vi "Corr Transducers To Meas Folder.vi"(8 "error in":errorcluster, 10 "measurement root path":path, 11 "transducers in":cluster{"channels":T1[], "last path":path} {"channels"."Phase index" min=1 step=1}) -> (0 "error out":errorcluster, 3 "transducers out":cluster{"channels":T1[], "last path":path} {"channels"."Phase index" min=1 step=1})   [LabVIEW 2013]
doc: "This VI will copy all transducer corrections to the measurement root path."
uses:
  Corr Tranducer Item.ctl
panel:
  # "ADC:"
  # "ADC:"
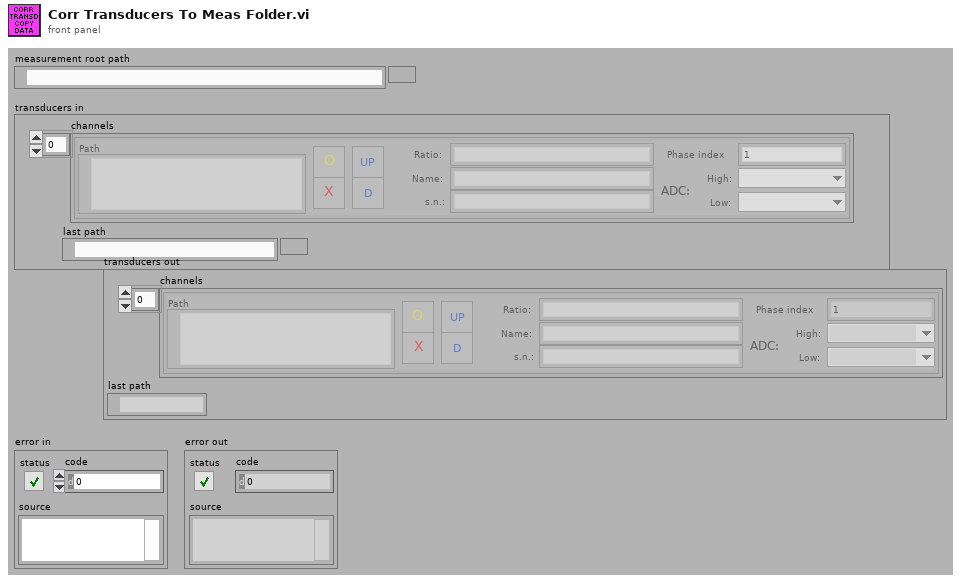
[diagram p1: front panel]
types:
  T1 = typedef "Corr Tranducer Item.ctl" = cluster{"Path":path, "Ratio:":string, "Name:":string, "btn rem":bool, "btn up":bool, "btn down":bool, "s.n.:":string, "btn open":bool, "ratio o/i":dbl, "chn hi":u16, "chn lo":u16, "Phase index":i32}
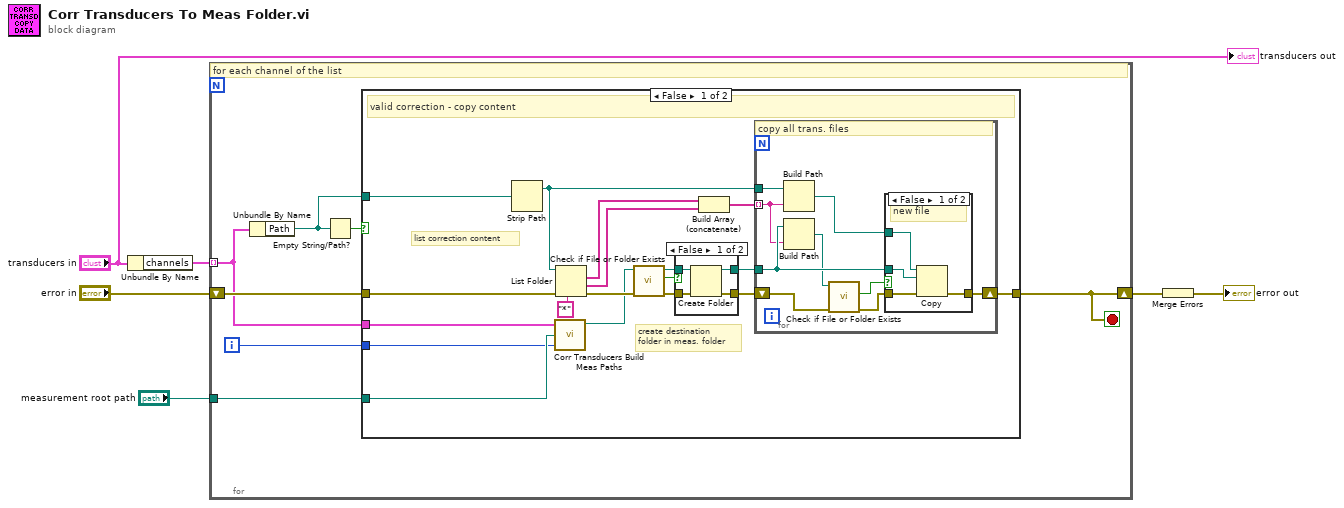
[diagram p0: block diagram]
diagram:
  n1 = Unbundle By Name("transducers in") -> ("channels"=w6:T1[])
  n2 = for {
    tunnel: w6 -> [w8] mode=indexing
    tunnel: "measurement root path" -> [w10]
    shift-right: [w9] -> w4
    shift-left: "error in" -> [w12]
    i -> [w7]
    stop <- w9 stop-if-true
    # "for each channel of the list"
    n3 = Unbundle By Name(w8) -> ("Path"=w11:path)
    n4 = Empty String/Path?(string/path=w11) -> (empty?=w13:bool)
    n5 = case shown="False" w13 {
      tunnel: w12 -> [w31 w52]
      tunnel: w11 -> [w23 _]
      tunnel: w10 -> [w21 _]
      tunnel: [w24 w52] -> w9
      tunnel: w8 -> [w22 _]
      tunnel: w7 -> [w14 _]
      frame False {
        # "create destination\nfolder in meas. folder"
        # "list correction content"
        # "valid correction - copy content"
        n6 = Strip Path(path=w23) -> (stripped path=w20:path)  [unwired: 1 out]
        n7 = call "Corr Transducers Build Meas Paths.vi"("transducer"=w22, "measurement folder root path"=w21, "transducer index"=w14) -> ("destination folder full path"=w17:path)  [unwired: 3 out]
        n8 = List Folder(path=w20, pattern="*", error in=w31) -> (filenames=w27:string[], folder names=w26:string[], error out=w19:errorcluster)  [unwired: 1 in, 1 out]
        n9 = call <vilib>:"Check if File or Folder Exists.vi"("error in (no error)"=w19, "path"=w17) -> ("error out"=w18:errorcluster, "file or folder exists?"=w15:bool, "dup path"=w16:path)  [unwired: 7 in]
        n10 = case shown="False" w15 {
          tunnel: [w35 w37] -> w29
          tunnel: [w34 w36] -> w28
          tunnel: w18 -> [w33 w37]
          tunnel: w16 -> [w32 w36]
          frame False {
            n11 = Create Folder(path (use dialog)=w32, error in=w33) -> (created path=w34:path, error out=w35:errorcluster)  [unwired: 1 in, 1 out]
          }
          frame True {
          }
        }
        n12 = Build Array (concatenate)(w27, w26) -> (w25:string[])
        n13 = for {
          tunnel: w28 -> [w42]
          shift-right: [w46] -> w24
          shift-left: w29 -> [w43]
          tunnel: w25 -> [w41] mode=indexing
          tunnel: w20 -> [w44]
          # "copy all trans. files"
          n14 = Build Path(base path=w44, name or relative path=w41) -> (appended path=w45:path)
          n15 = Build Path(base path=w42, name or relative path=w41) -> (appended path=w40:path)
          n16 = call <vilib>:"Check if File or Folder Exists.vi"("error in (no error)"=w43, "path"=w40) -> ("error out"=w38:errorcluster, "file or folder exists?"=w39:bool)  [unwired: 7 in, 1 out]
          n17 = case shown="False" w39 {
            tunnel: w38 -> [w50 w51]
            tunnel: [w49 w51] -> w46
            tunnel: w42 -> [w48 _]
            tunnel: w45 -> [w47 _]
            frame False {
              # "new file"
              n18 = Copy(8:w50, 10:w48, 11:w47) -> (0:w49:errorcluster)  [unwired: 2 in, 2 out]
            }
            frame True {
              # "skip if file\nalready there"
            }
          }
        }
      }
      frame True {
      }
    }
  }
  n19 = Merge Errors(w4) -> (→"error out":errorcluster)
  "transducers out" <- "transducers in"
